vi "SFM-Create (continuous).vi"(0 "New":T1, 5 "Old":T1, 7 "Fs (Hz)":dbl=100000.0, 9 "Npts":i32) -> (4 "Out":T1, 8 "Y":dbl[](array[numeric]))   [LabVIEW 2015]
uses:
  SFM-Params.ctl
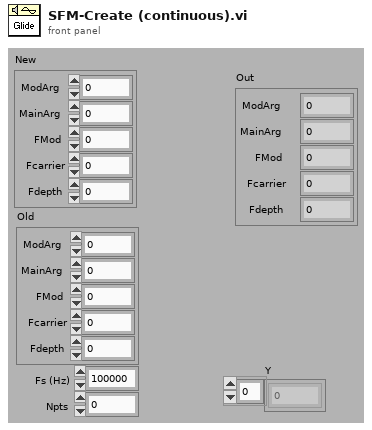
[diagram p1: front panel]
types:
  T1 = typedef "SFM-Params.ctl" = cluster{"ModArg":dbl, "MainArg":dbl, "FMod":dbl, "Fcarrier":dbl, "Fdepth":dbl}
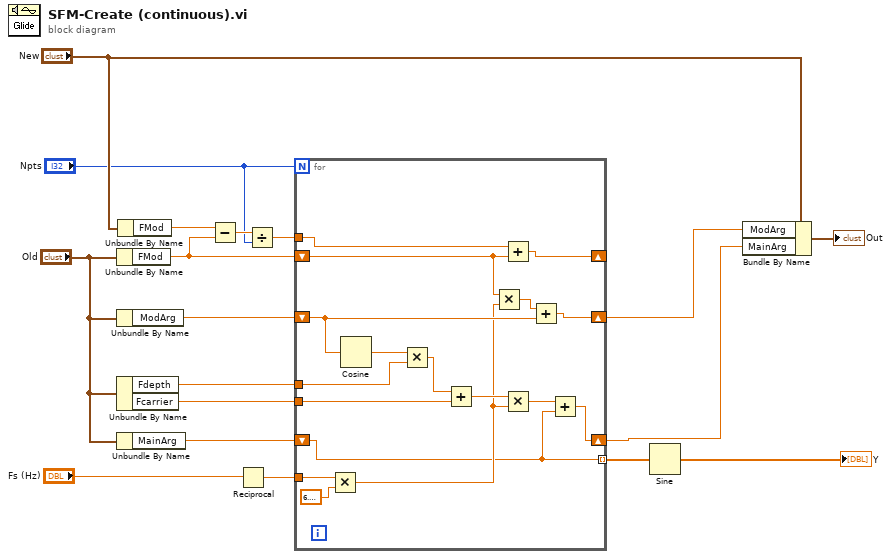
[diagram p0: block diagram]
diagram:
  n1 = Unbundle By Name("Old") -> ("FMod"=w11:dbl)
  n2 = Unbundle By Name("Old") -> ("ModArg"=w6:dbl)
  n3 = Unbundle By Name("Old") -> ("Fdepth"=w10:dbl, "Fcarrier"=w9:dbl)
  n4 = Unbundle By Name("Old") -> ("MainArg"=w4:dbl)
  n5 = Unbundle By Name("New") -> ("FMod"=w1:dbl)
  n6 = Subtract(x=w1, y=w11) -> (x-y=w16:dbl)
  n7 = Reciprocal(x="Fs (Hz)") -> (1/x=w12:dbl)
  n8 = Divide(x=w16, y="Npts") -> (x/y=w8:dbl)
  n9 = for {
    N: "Npts" -> [_]
    tunnel: w12 -> [w28]
    shift-right: [w29] -> w14
    shift-left: w6 -> [w31]
    tunnel: w8 -> [w22]
    tunnel: w10 -> [w33]
    tunnel: w9 -> [w32]
    shift-right: [w20] -> w2
    shift-left: w4 -> [w19]
    tunnel: [w19] -> w3 mode=indexing
    shift-right: [w21] -> _
    shift-left: w11 -> [w23]
    n10 = Multiply(x=w28, y=6.283185307179586) -> (x*y=w25:dbl)
    n11 = Cosine(x=w31) -> (cos(x)=w35:dbl)
    n12 = Multiply(x=w35, y=w33) -> (x*y=w34:dbl)
    n13 = Add(x=w34, y=w32) -> (x+y=w26:dbl)
    n14 = Multiply(x=w23, y=w25) -> (x*y=w30:dbl)
    n15 = Add(x=w22, y=w23) -> (x+y=w21:dbl)
    n16 = Multiply(x=w26, y=w25) -> (x*y=w24:dbl)
    n17 = Add(x=w30, y=w31) -> (x+y=w29:dbl)
    n18 = Add(x=w24, y=w19) -> (x+y=w20:dbl)
  }
  n19 = Sine(x=w3) -> (sin(x)=→"Y":dbl[])
  n20 = Bundle By Name(cluster="New", "ModArg"=w14, "MainArg"=w2) -> (→"Out":T1)
